vi "PathFlagConst.vi"() -> (3 "路径":path)   [LabVIEW 2016, in "PanelRootNode.lvclass"]
uses:
  PanelRootNode.lvclass
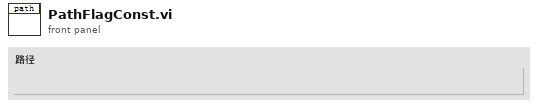
[diagram p1: front panel]
types:
  T1 = enum32{"invalid app kind", "Development System", "Run Time System", "Student Edition", "Embedded LabVIEW", "Evaluation", "Custom"}
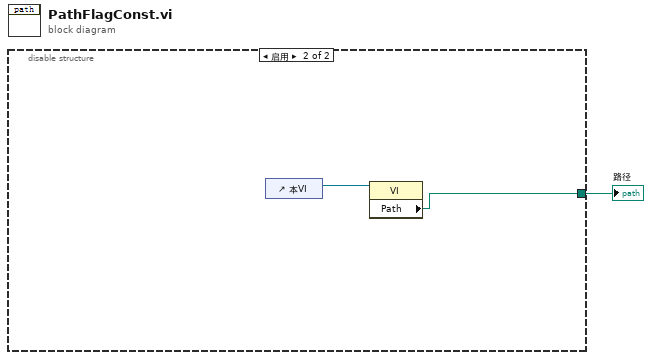
[diagram p0: block diagram]
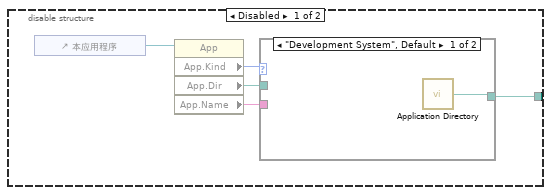
[diagram p2: hidden frame]
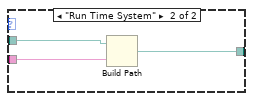
[diagram p3: hidden frame]
diagram:
  n1 = disable-structure shown="启用" {
    disable-tunnel: [w4 w11] -> w1
    frame Disabled {
      n2 = control-ref of="本应用程序"() -> (w6:refnum<vi>)
      n3 = property class="App"(reference=w6) -> ("App.Kind"=w2:T1, "App.Dir"=w3:path, "App.Name"=w5:string)  [unwired: 1 in, 2 out]
      n4 = case shown="\"Development System\", Default" w2 {
        tunnel: w5 -> [_ w10]
        tunnel: [w7 w9] -> w4
        tunnel: w3 -> [_ w8]
        frame "Development System", Default {
          n5 = call <vilib>:"Application Directory.vi"() -> ("Application Directory"=w7:path)
        }
        frame "Run Time System" {
          n6 = Build Path(base path=w8, name or relative path=w10) -> (appended path=w9:path)
        }
      }
    }
    frame Enabled {
      n7 = control-ref of="本VI"() -> (w12:refnum<vi>)
      n8 = property class="VI"(reference=w12) -> ("Path"=w11:path)  [unwired: 1 in, 2 out]
    }
  }
  "路径" <- w1
